vi "SDG60ConfArbWaveform1.vi"(5 "Select Channel (1:Channel 1)":i32(ring)=1 items=["Channel 1"=1, "Channel 2"=2], 6 "DC Offset (0.00 V)":dbl min=-10.0 max=10.0, 7 "Amplitude (1.0 Vpp)":dbl=1.0 min=0.001 max=20.0 step=1.0 format="%#.3f", 8 "error in (no error)":errorcluster, 9 "Phase (0.0 degrees)":dbl=0.002 min=-360.0 max=360.0 format="%#.1g", 10 "Frequency (1000 Hz)":dbl=1000.0 min=1e-06 max=160000000.0 step=1.0 format="%#.6g", 11 "VISA resource name":refnum<visa-resource-name>="USB0::0xF4EC::0x1101::SDG6XEBC5R0119::INSTR") -> ()   [LabVIEW 2018]
doc: "Sets the waveform parameters for an arbitrary waveform. This VI should be called after <b>Create Arbitrary Waveform.vi</b> (for user defined arbitrary waveform) and <b>Select Arbitrary Waveform.vi</b>"
panel:
  out "error out":errorcluster
  out "VISA resource name out":refnum<visa-resource-name>
  in  "DDS/TArb 0: DDS":u16(ring) items=["DDS", "TrueArb"]
  in  "Interpolation 0: Zero-order":u16(ring) items=["Zero-Order", "Linear"]
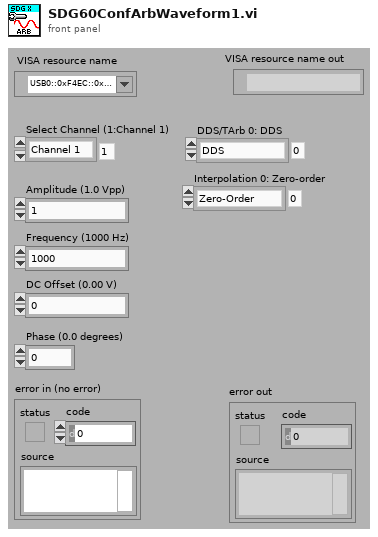
[diagram p1: front panel]
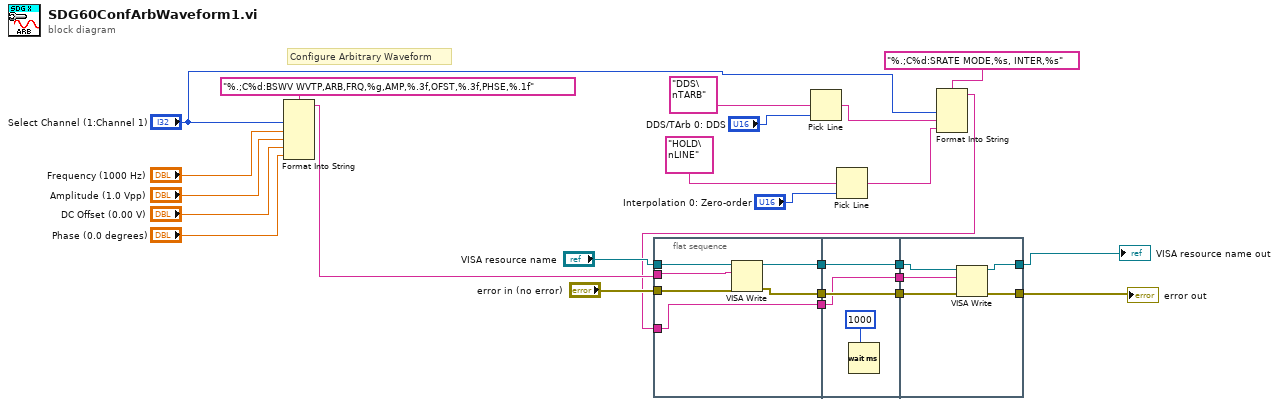
[diagram p0: block diagram]
diagram:
  # "Configure Arbitrary Waveform"
  n1 = Format Into String(format string="%.;C%d:BSWV WVTP,ARB,FRQ,%g,AMP,%.3f,OFST,%.3f,PHSE,%.1f", "Select Channel (1:Channel 1)", "Frequency (1000 Hz)", "Amplitude (1.0 Vpp)", "DC Offset (0.00 V)", "Phase (0.0 degrees)") -> (resulting string=w9:string)  [unwired: 2 in, 1 out]
  n2 = flat-sequence {
    tunnel: [w29] -> w12
    tunnel: "VISA resource name" -> [w31]
    tunnel: w9 -> [w30]
    tunnel: "error in (no error)" -> [w28]
    tunnel: [w27] -> w5
    tunnel: w3 -> [w26]
    tunnel: [w26] -> w2
    tunnel: w12 -> [w34]
    tunnel: [w34] -> w11
    tunnel: [w33] -> w6
    tunnel: w5 -> [w33]
    tunnel: w2 -> [w32]
    tunnel: [w32] -> w1
    tunnel: [w36] -> w10
    tunnel: w11 -> [w37]
    tunnel: w6 -> [w40]
    tunnel: [w39] -> w4
    tunnel: w1 -> [w38]
    frame #0 {
      n3 = VISA Write(VISA resource name=w31, write buffer=w30, error in (no error)=w28) -> (VISA resource name out=w29:refnum<visa-resource-name>, error out=w27:errorcluster)  [unwired: 1 out]
    }
    frame #1 {
      n4 = Wait (ms)(milliseconds to wait=1000 ("x")) -> ()  [unwired: 1 out]
    }
    frame #2 {
      n5 = VISA Write(VISA resource name=w37, write buffer=w38, error in (no error)=w40) -> (VISA resource name out=w36:refnum<visa-resource-name>, error out=w39:errorcluster)  [unwired: 1 out]
    }
  }
  n6 = Pick Line(multi-line string="DDS\nTARB", line index="DDS/TArb 0: DDS") -> (output string=w14:string)  [unwired: 1 in]
  n7 = Pick Line(multi-line string="HOLD\nLINE", line index="Interpolation 0: Zero-order") -> (output string=w17:string)  [unwired: 1 in]
  n8 = Format Into String(format string="%.;C%d:SRATE MODE,%s, INTER,%s", "Select Channel (1:Channel 1)", w14, w17) -> (resulting string=w3:string)  [unwired: 2 in, 1 out]
  "VISA resource name out" <- w10
  "error out" <- w4
